vi "Set TableName.vi"(8 "error in (no error)":errorcluster caption="entrée d'erreur (pas d'erreur)", 10 "TableName":string, 11 "Database Drivers en entrée":refnum<class "Database Drivers.lvclass">) -> (0 "error out":errorcluster caption="sortie d'erreur", 3 "Database Drivers en sortie":refnum<class "Database Drivers.lvclass">)   [LabVIEW 2020, in "Library Instrument & Equipement.lvlib" / "Library Database.lvlib" / "Database Drivers.lvclass"]
uses:
  Database Drivers.lvclass
  Database Drivers.lvclass/Database Drivers.ctl
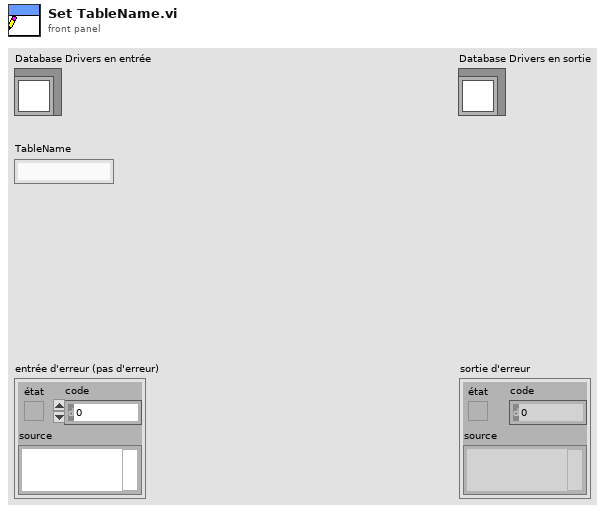
[diagram p1: front panel]
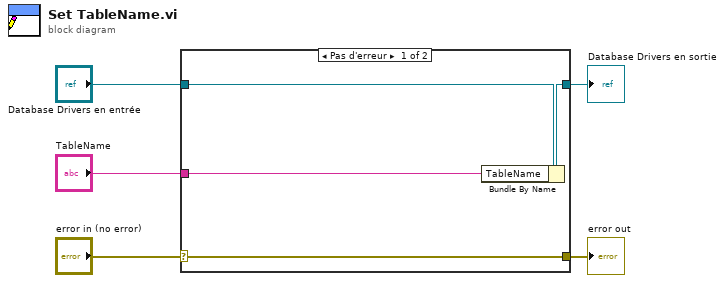
[diagram p0: block diagram]
diagram:
  n1 = case shown="Pas d'erreur" "error in (no error)" {
    selector: "error in (no error)" -> [w9 w10]
    tunnel: [w9 w10] -> w4
    tunnel: [w7 w11] -> w2
    tunnel: "Database Drivers en entrée" -> [w8 w11]
    tunnel: "TableName" -> [w6 _]
    frame No Error {
      n2 = Bundle By Name(cluster=w8, "TableName"=w6) -> (w7:refnum<class "Database Drivers.lvclass">)
    }
    frame Error {
    }
  }
  "error out" <- w4
  "Database Drivers en sortie" <- w2
